vi "Initialize.vi"(8 "error in (no error)":errorcluster, 11 "PowerSupply in":refnum<class "PowerSupply.lvclass">) -> (0 "error out":errorcluster, 3 "PowerSupply out":refnum<class "PowerSupply.lvclass">)   [LabVIEW 2020, in "PowerSupply.lvclass"]
uses:
  PowerSupply.lvclass
  PowerSupply.lvclass/PowerSupply.ctl
  <vilib>/DigilentWF/DigilentWF.lvlib
panel:
  in  "Device Name":string
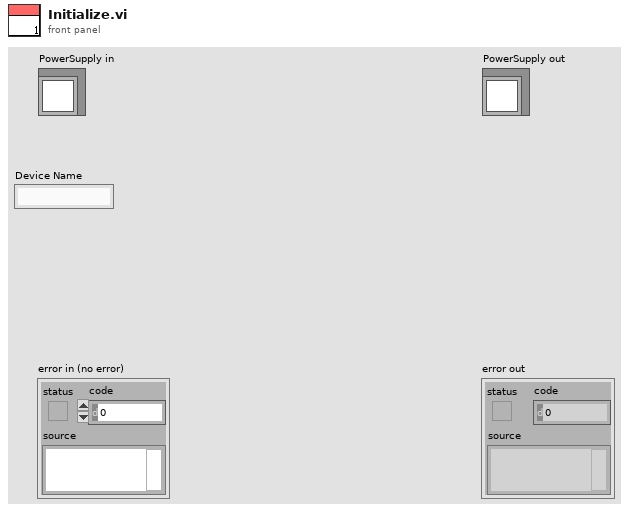
[diagram p1: front panel]
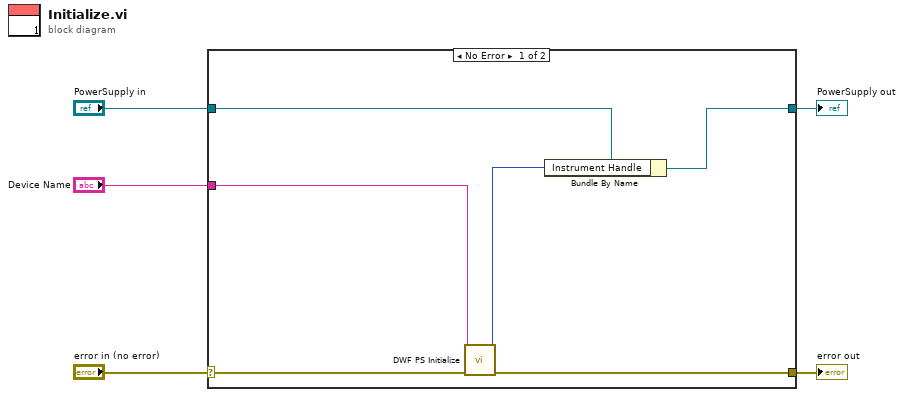
[diagram p0: block diagram]
diagram:
  n1 = case shown="No Error" "error in (no error)" {
    selector: "error in (no error)" -> [w10 w13]
    tunnel: [w9 w13] -> w4
    tunnel: [w7 w12] -> w2
    tunnel: "PowerSupply in" -> [w8 w12]
    tunnel: "Device Name" -> [w11 _]
    frame No Error {
      n2 = call <vilib>:"DWF PS Initialize.vi"("Device Name"=w11, "Error In"=w10) -> ("Instrument Handle Out"=w6:u32, "Error Out"=w9:errorcluster)  [unwired: 12 in]
      n3 = Bundle By Name(cluster=w8, "Instrument Handle"=w6) -> (w7:refnum<class "PowerSupply.lvclass">)
    }
    frame Error {
    }
  }
  "error out" <- w4
  "PowerSupply out" <- w2
